vi "Measure.vi"(4 "new data?":bool, 5 "position or angle":enum16{"position", "angle"}(ring), 6 "reset?":bool, 7 "nominal radius":dbl, 8 "position":u32, 9 "angle":dbl) -> (0 "data":cluster{dbl[], dbl[]}, 1 "count":u32, 2 "instant values":T1, 3 "time step":dbl)   [LabVIEW 2011]
doc: "Reads from the RadialValue shared variable the current radial position measured by the linear displacement gauge and gives the instant values cluster (measurement , mean value, and st.dev.), and keeps a buffer containing all the (angle,position) values since the last time that the reset? input was true.\n\nSince the RadialValue could be updated more often than the angular position, this VI performs a point-by-point mean and st.dev. calculation, resetting the buffer every time that a new angular position is reached. In this way, each (angle,radius) point is the average of all the measurements collected at the same angular position."
uses:
  <vilib>/ptbypt/NI_PtbyPt.lvlib
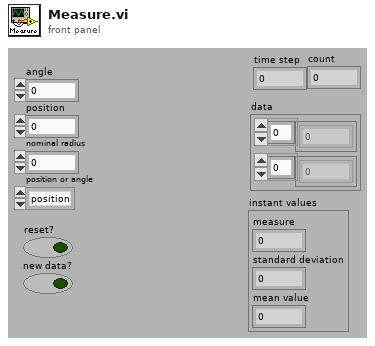
[diagram p1: front panel]
types:
  T1 = cluster{"measure":dbl, "standard deviation":dbl, "mean value":dbl}
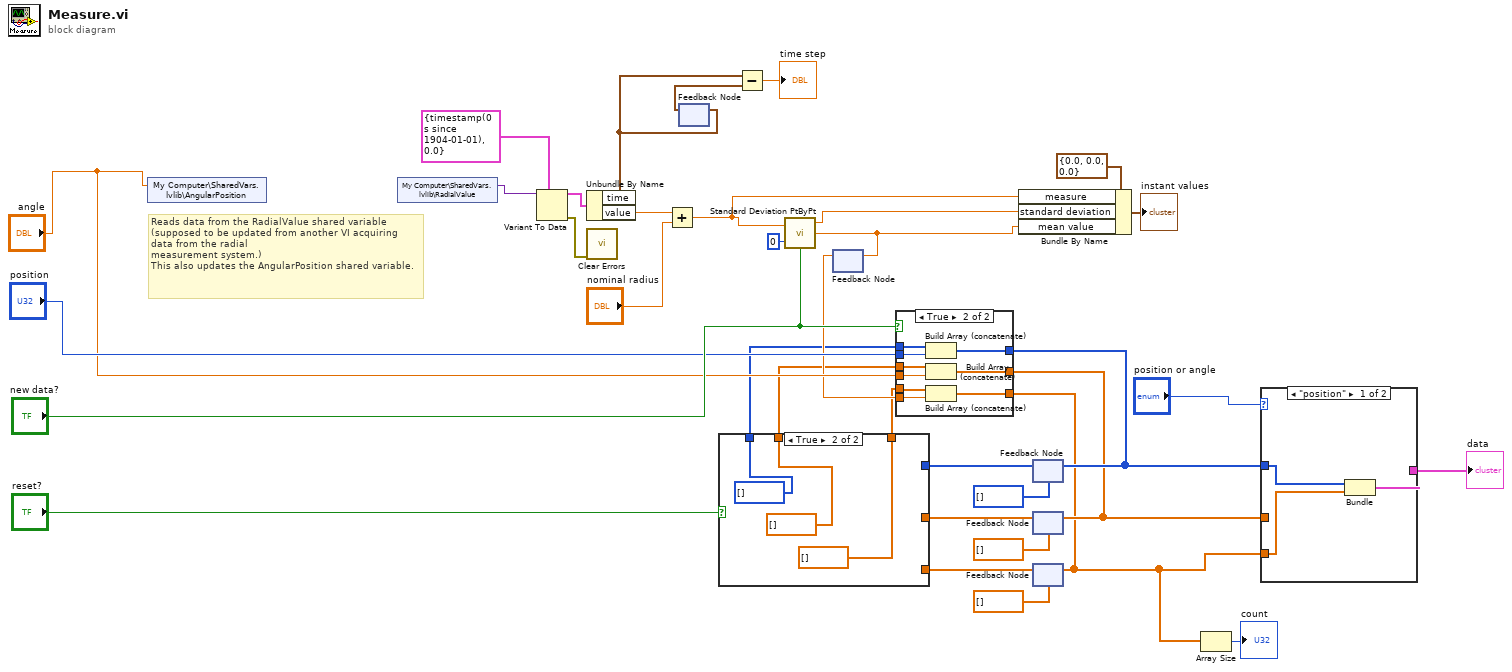
[diagram p0: block diagram]
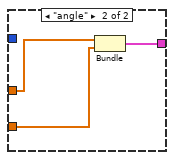
[diagram p2: hidden frame]
diagram:
  # "Reads data from the RadialValue shared variable\n(supposed to be updated from another VI acquiring data from the radial\nmeasurement system.)\nThis also updates the AngularPosition shared variable."
  n1 = shared-variable "My Computer\\SharedVars.lvlib\\AngularPosition"("angle") -> ()  [unwired: 1 in, 1 out]
  n2 = shared-variable "My Computer\\SharedVars.lvlib\\RadialValue"() -> (w16:variant)  [unwired: 1 in, 1 out]
  n3 = Variant To Data(type=cluster{"time":timestamp, "value":dbl} {"time"=timestamp(0 s since 1904-01-01), "value"=0.0} ("input cluster"), Variant=w16) -> (data=w14:cluster{"time":timestamp, "value":dbl}, error out=w6:errorcluster)  [unwired: 1 in]
  n4 = Unbundle By Name(w14) -> ("time"=w9:timestamp, "value"=w2:dbl)
  n5 = call <vilib>:"Clear Errors.vi"("error in (no error)"=w6) -> ()  [unwired: 6 in, 1 out]
  n6 = Add(x=w2, y="nominal radius") -> (x+y=w1:dbl)
  n7 = feedback #1() -> (w8:timestamp)  [unwired: 1 in]
  n8 = feedback-in #1(w9) -> ()
  n9 = Subtract(x=w9, y=w8) -> (x-y=→"time step":dbl)
  n10 = call <vilib>:"Standard Deviation PtByPt.vi"("x"=w1, "sample length"=0, "initialize"="new data?") -> ("standard deviation"=w11:dbl, "mean"=w10:dbl)  [unwired: 1 out]
  n11 = feedback #2() -> (w31:dbl)  [unwired: 1 in]
  n12 = feedback-in #2(w10) -> ()
  n13 = Bundle By Name(cluster=T1 {"measure"=0.0, "standard deviation"=0.0, "mean value"=0.0}, "measure"=w1, "standard deviation"=w11, "mean value"=w10) -> (→"instant values":T1)
  n14 = feedback #3(u32[] []) -> (w23:u32[])
  n15 = feedback #4(dbl[] []) -> (w24:dbl[])
  n16 = feedback #5(dbl[] []) -> (w27:dbl[])
  n17 = case shown="True" "reset?" {
    tunnel: w27 -> [w36 _]
    tunnel: [w36 dbl[] []] -> w26
    tunnel: [w38 dbl[] []] -> w25
    tunnel: w24 -> [w38 _]
    tunnel: w23 -> [w37 _]
    tunnel: [w37 u32[] []] -> w22
    frame False {
    }
    frame True {
    }
  }
  n18 = case shown="True" "new data?" {
    tunnel: "position" -> [_ w53]
    tunnel: w25 -> [w43 w49]
    tunnel: w22 -> [w44 w52]
    tunnel: w26 -> [w42 w51]
    tunnel: "angle" -> [_ w50]
    tunnel: w31 -> [_ w48]
    tunnel: [w44 w47] -> w19
    tunnel: [w43 w46] -> w18
    tunnel: [w42 w45] -> w5
    frame False {
    }
    frame True {
      n19 = Build Array (concatenate)(w52, w53) -> (w47:u32[])
      n20 = Build Array (concatenate)(w49, w50) -> (w46:dbl[])
      n21 = Build Array (concatenate)(w51, w48) -> (w45:dbl[])
    }
  }
  n22 = feedback-in #3(w19) -> ()
  n23 = feedback-in #4(w18) -> ()
  n24 = feedback-in #5(w5) -> ()
  n25 = Array Size(array=w5) -> (size(s)=→"count":i32)
  n26 = case shown="\"position\"" "position or angle" {
    tunnel: w19 -> [w56 _]
    tunnel: w18 -> [_ w59]
    tunnel: w5 -> [w55 w58]
    tunnel: [w54 w57] -> w17
    frame "position" {
      n27 = Bundle(w56, w55) -> (w54:cluster{u32[], dbl[]})  [unwired: 1 in]
    }
    frame "angle" {
      n28 = Bundle(w59, w58) -> (w57:cluster{dbl[], dbl[]})  [unwired: 1 in]
    }
  }
  "data" <- w17
